vi "TestLibGetChecksumFile.vi"() -> ()   [LabVIEW 2020]
uses:
  LabviewTools32.dll
panel:
  out "Array":T1(array[cluster]) {"vChecksumReference" format="%04x"; "vChecksumCalculated" format="%04x"}
  in  "Path":path=path "P:/Meetdata/SapDwh/Mrc"
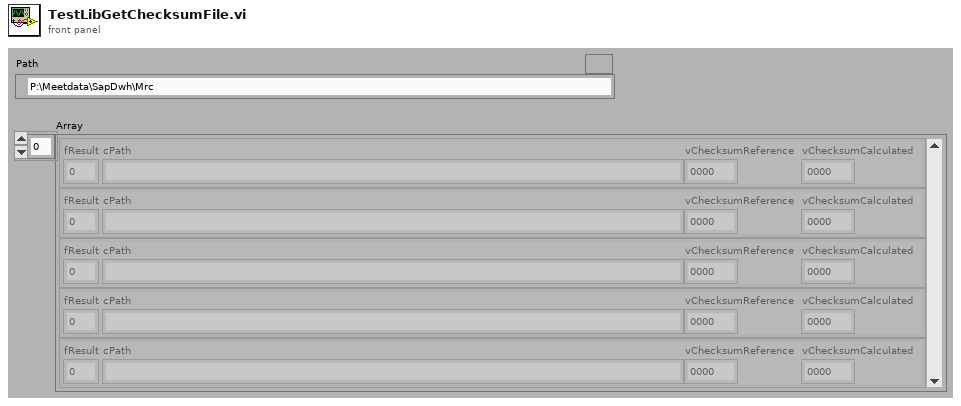
[diagram p1: front panel]
types:
  T1 = cluster{"fResult":i32, "cPath":string, "vChecksumReference":u16, "vChecksumCalculated":u16}[]
  T2 = cluster{"fResult":i32, "cFilePath":string, "vReferenceChecksum":u16, "vCalculatedChecksum":u16}
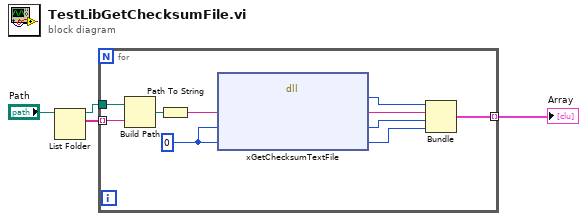
[diagram p0: block diagram]
diagram:
  n1 = List Folder(path="Path") -> (path out=w2:path, filenames=w3:string[])  [unwired: 3 in, 2 out]
  n2 = for {
    tunnel: w3 -> [w11] mode=indexing
    tunnel: w2 -> [w13]
    tunnel: [w9] -> w1 mode=indexing
    w5 = u16 0
    n3 = Build Path(base path=w13, name or relative path=w11) -> (appended path=w12:path)
    n4 = Path To String(path=w12) -> (string=w14:string)
    n5 = dll-call lib="C:/Factory/FactoryGenericTools/Dll/LabviewTools32.dll" fn="xGetChecksumTextFile"("cFilePath"=w14, "vReferenceChecksum"=w5, "vCalculatedChecksum"=w5) -> ("fResult"=w7:i32, "cFilePath"=w10:string, "vReferenceChecksum"=w8:u16, "vCalculatedChecksum"=w6:u16)  [unwired: 3 in, 2 out]
    n6 = Bundle("fResult"=w7, "cFilePath"=w10, "vReferenceChecksum"=w8, "vCalculatedChecksum"=w6) -> (w9:T2)  [unwired: 1 in]
  }
  "Array" <- w1
